vi "Pointer producer consumer Cloud Detector.vi"(8 "Real-time Values":dbl[](array[numeric]), 10 "Cloud Sensitivity":i8, 11 "Cloud Ctrl":bool) -> (3 "Cloud Detector":bool)   [LabVIEW 2014]
panel:
  out "CD_User":i16
  out "CD_Act":i16
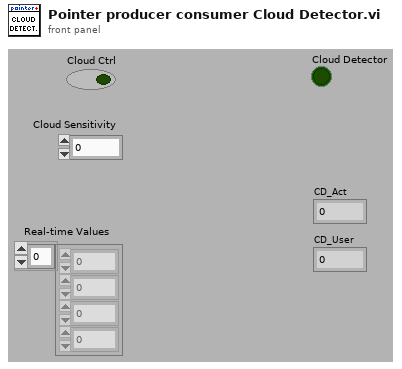
[diagram p1: front panel]
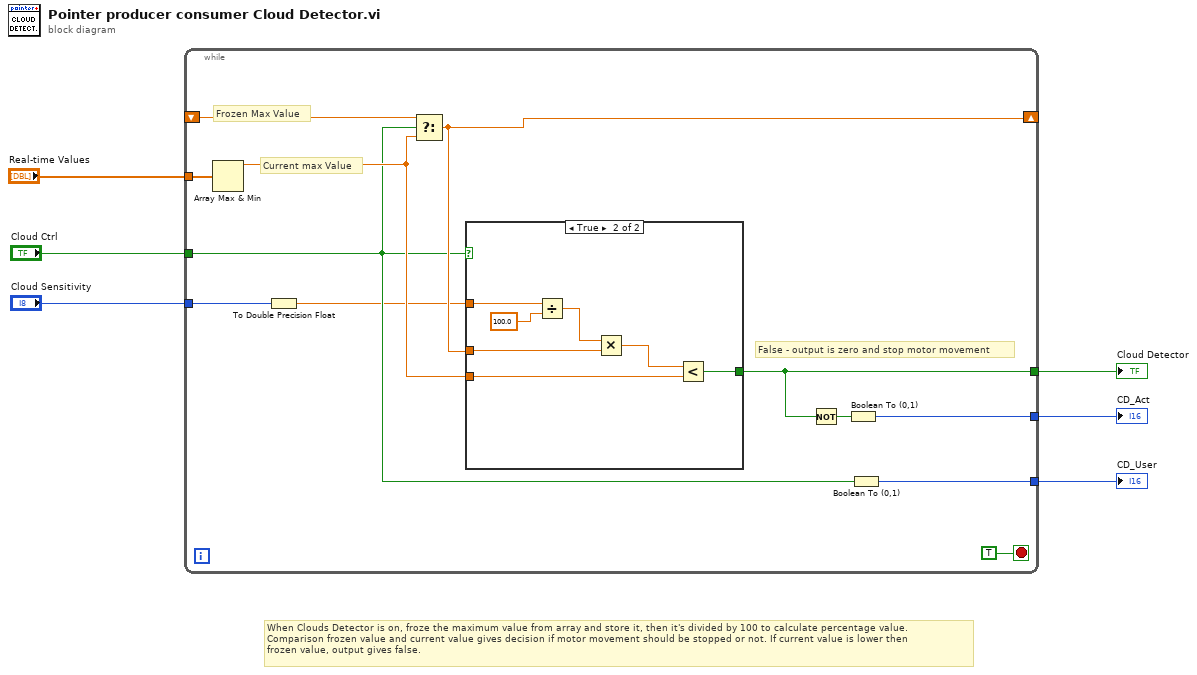
[diagram p0: block diagram]
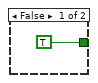
[diagram p2: hidden frame]
diagram:
  # "When Clouds Detector is on, froze the maximum value from array and store it, then it's divided by 100 to calculate percentage value. \nComparison frozen value and current value gives decision if motor movement should be stopped or not. If current value is lower then \nfrozen value, output gives false."
  n1 = while {
    tunnel: [w17] -> w5
    tunnel: [w16] -> w4
    tunnel: "Cloud Sensitivity" -> [w8]
    tunnel: "Cloud Ctrl" -> [w9]
    tunnel: [w18] -> w6
    tunnel: "Real-time Values" -> [w13]
    shift-right: [w10] -> _
    shift-left: _ -> [w12]
    stop <- TRUE stop-if-true
    # "Current max Value"
    # "Frozen Max Value"
    # "False - output is zero and stop motor movement"
    n2 = Array Max & Min(array=w13) -> (max value=w11:dbl)  [unwired: 3 out]
    n3 = To Double Precision Float(number=w8) -> (double precision float=w7:dbl)
    n4 = Select(t=w12, s=w9, f=w11) -> (s? t:f=w10:dbl)
    n5 = case shown="True" w9 {
      tunnel: w7 -> [_ w26]
      tunnel: w10 -> [_ w23]
      tunnel: w11 -> [_ w20]
      tunnel: [TRUE w21] -> w18
      frame False {
      }
      frame True {
        n6 = Divide(x=w26, y=100.0) -> (x/y=w24:dbl)
        n7 = Multiply(x=w24, y=w23) -> (x*y=w22:dbl)
        n8 = Less?(x=w22, y=w20) -> (x < y?=w21:bool)
      }
    }
    n9 = Not(x=w18) -> (.not. x?=w15:bool)
    n10 = Boolean To (0,1)(Boolean=w15) -> (0, 1=w17:i16)
    n11 = Boolean To (0,1)(Boolean=w9) -> (0, 1=w16:i16)
  }
  "Cloud Detector" <- w6
  "CD_Act" <- w5
  "CD_User" <- w4
